vi "_IP Reporter.vi"(4 "ignore Gateway IP?(T)":bool=TRUE, 6 "Load From File(F)":bool, 8 "error in":errorcluster, 9 "notifier":refnum<notifier>, 10 "Init-Information":string, 11 "Setttings":T1={"address"="234.5.6.7", "receiver port"=58432, "Ignore Gateway IP"=TRUE, "HostName"=""}) -> (0 "error out":errorcluster)   [LabVIEW 2017]
doc: "Creates a write-only UDP multicast session and sends data to the specified port."
uses:
  _Typedef/Def-IniSettings -- Cluster.ctl
  _Typedef/Def-Report -- Cluster.ctl
  d1e7c7ed-84d8-4585-9177-9cc17e079b9e.vi
  <vilib>/Utility/error.llb/Clear Errors.vi
  d1e7c7ed-84d8-4585-9177-9cc17e079b9e.vi/c738ad2c-660d-48ef-8aa3-24bba17e300f.vi
  <vilib>/Utility/libraryn.llb/Recursive File List.vi
  <vilib>/Utility/config.llb/Open Config Data.vi
  <userlib>/_OpenG.lib/lvdata/lvdata.llb/Get Data Name__ogtk.vi
  <vilib>/Utility/config.llb/Get Section Names.vi
  <userlib>/_OpenG.lib/variantconfig/variantconfig.llb/Write Section Cluster__ogtk.vi
  <userlib>/_OpenG.lib/variantconfig/variantconfig.llb/Read Section Cluster__ogtk.vi
  <vilib>/Utility/config.llb/Close Config Data.vi
  <vilib>/Utility/tcp.llb/UDP Multicast Write-Only Open.vi
panel:
  out "JSON string":string
  in  "Stop":bool
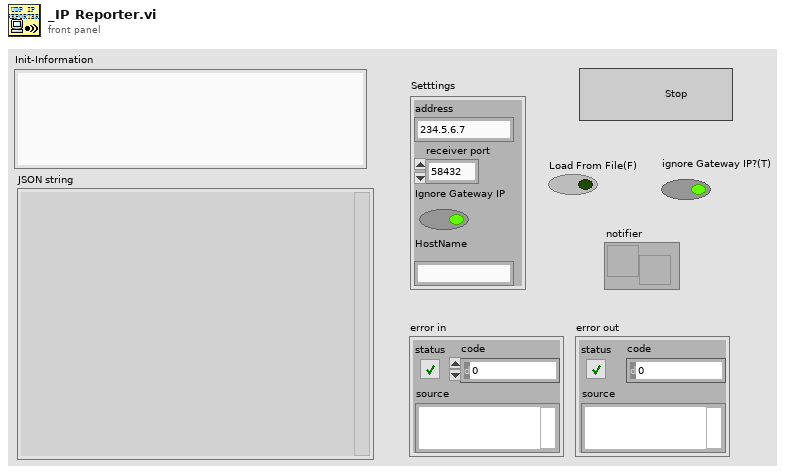
[diagram p1: front panel]
types:
  T1 = typedef "Def-IniSettings -- Cluster.ctl" = cluster{"address":string, "receiver port":u16, "Ignore Gateway IP":bool, "HostName":string}
  T2 = typedef "Def-Report -- Cluster.ctl" = cluster{"Host Name":string, "IPs":string[], "Timestamp":string, "Information":string}
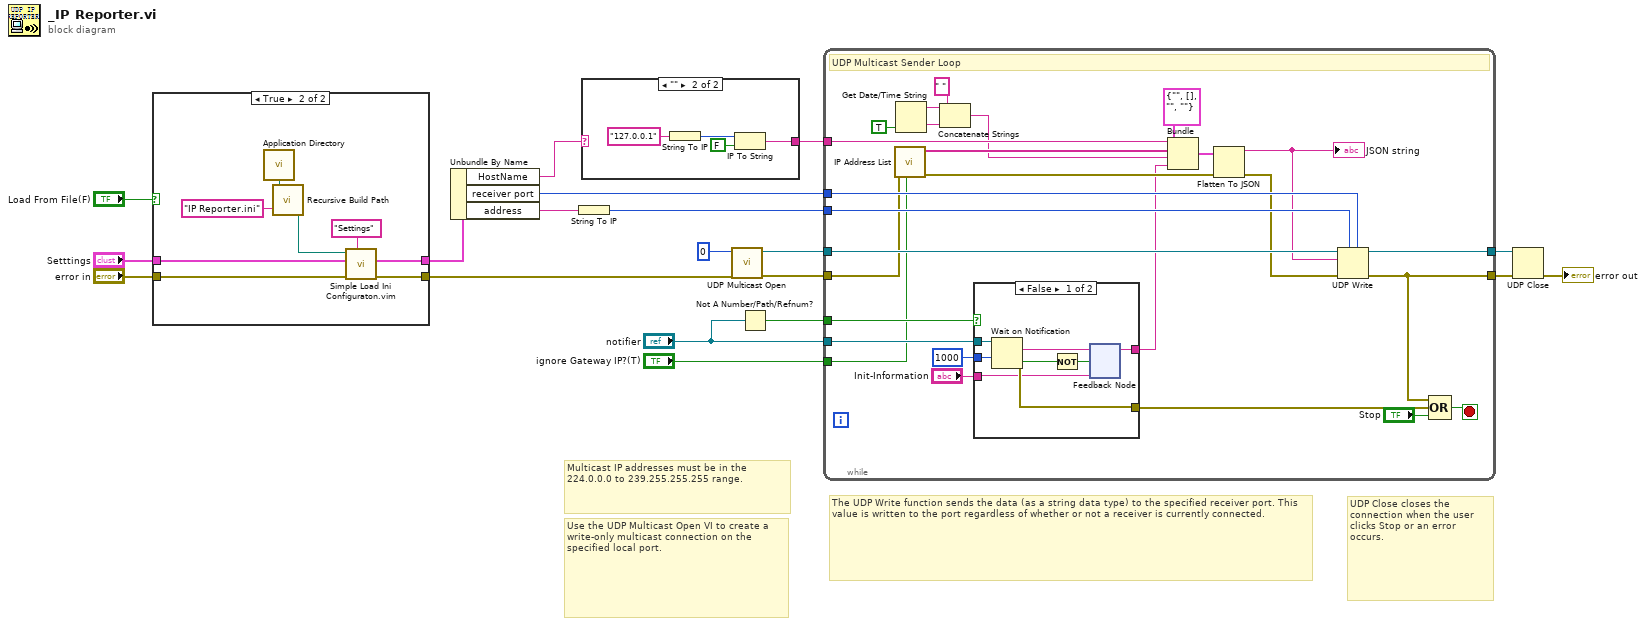
[diagram p0: block diagram]
diagram:
  # "UDP Close closes the connection when the user clicks Stop or an error occurs."
  # "Multicast IP addresses must be in the 224.0.0.0 to 239.255.255.255 range."
  # "The UDP Write function sends the data (as a string data type) to the specified receiver port. This value is written to the port regardless of whether or not a receiver is currently connected."
  # "Use the UDP Multicast Open VI to create a write-only multicast connection on the specified local port."
  n1 = case shown="True" "Load From File(F)" {
    tunnel: [w21 w29] -> w14
    tunnel: [w20 w28] -> w12
    tunnel: "Setttings" -> [w21 w24]
    tunnel: "error in" -> [w20 w23]
    frame False {
    }
    frame True {
      n2 = call <vilib>:"Application Directory.vi"() -> ("Application Directory"=w27:path)
      n3 = call "Recursive Build Path.vi"("file name"="IP Reporter.ini", "Path"=w27) -> ("file path name"=w25:path)  [unwired: 1 in]
      n4 = call "Simple Load Ini Configuraton.vim"("Session"="Settings", "error in (no error)"=w23, "Default Settings"=w24, "file path name"=w25) -> ("error out"=w28:errorcluster, "Settings out"=w29:T1)  [unwired: 6 in]
    }
  }
  n5 = Unbundle By Name(w14) -> ("HostName"=w9:string, "receiver port"=w11:u16, "address"=w13:string)
  n6 = String To IP(1:w13) -> (0:w17:u32)
  n7 = case shown="\"\"" w9 {
    selector: w9 -> [w30 _]
    tunnel: [w30 w34] -> w10
    frame "False", Default {
    }
    frame "" {
      n8 = String To IP(1:"127.0.0.1" ("name")) -> (0:w33:u32)
      n9 = IP To String(1:FALSE ("dot notation? (F)"), 2:w33) -> (0:w34:string)
    }
  }
  n10 = call-poly <vilib>:"UDP Multicast Open.vi"("error in (no error)"=w12, "port"=u16 0) -> ("error out"=w15:errorcluster, "connection ID"=w16:refnum<k16>)  [unwired: 8 in]
  n11 = Not A Number/Path/Refnum?(number/path/refnum="notifier") -> (NaN/Path/Refnum?=w7:bool)
  n12 = while {
    tunnel: [w43] -> w18
    tunnel: w16 -> [w61]
    tunnel: w15 -> [w55]
    tunnel: [w58] -> w19
    tunnel: w17 -> [w57]
    tunnel: w11 -> [w56]
    tunnel: w10 -> [w48]
    tunnel: "notifier" -> [w47]
    tunnel: w7 -> [w44]
    tunnel: "ignore Gateway IP?(T)" -> [w37]
    stop <- w60 stop-if-true
    # "UDP Multicast Sender Loop"
    n13 = call "IP Address List.vi"("ignore Gateway IP?"=w37, "error in (no error)"=w55) -> ("error out"=w54:errorcluster, "Array"=w50:string[])  [unwired: 8 in]
    n14 = Get Date/Time String(want seconds? (F)=TRUE) -> (date string=w42:string, time string=w41:string)  [unwired: 2 in]
    n15 = Concatenate Strings(w42, " " ("string"), w41) -> (w39:string)
    n16 = case shown="False" w44 {
      tunnel: w47 -> [w69 _]
      tunnel: 1000 ("timeout in ms (-1)") -> [w68 _]
      tunnel: [w67 _] -> w45
      tunnel: [w63 w70] -> w36
      tunnel: "Init-Information" -> [w62 w70]
      frame False {
        n17 = Wait on Notification(notifier=w69, timeout in ms (-1)=w68) -> (notification=w65:string, timed out?=w66:bool, error out=w67:errorcluster)  [unwired: 2 in, 1 out]
        n18 = Not(x=w66) -> (.not. x?=w64:bool)
        n19 = feedback-in #1(w65, w64) -> ()
        n20 = feedback #1(w62) -> (w63:string)
      }
      frame True {
      }
    }
    n21 = Bundle(cluster=T2 {"Host Name"="", "IPs"=[], "Timestamp"="", "Information"=""} ("Pack"), "Host Name"=w48, "IPs"=w50, "Timestamp"=w39, "Information"=w36) -> (w49:T2)
    n22 = Flatten To JSON(anything=w49, error in (no error)=w54) -> (JSON string=w52:string, 11:w53:errorcluster)  [unwired: 1 in]
    "JSON string" <- w52
    n23 = UDP Write(address=w57, port or service name=w56, connection ID=w61, data in=w52, 8:w53) -> (error out=w43:errorcluster, 3:w58:refnum<k16>)  [unwired: 1 in]
    n24 = Compound Arithmetic op=OR(w43, w45, "Stop") -> (w60:bool)
  }
  n25 = UDP Close(connection ID=w19, 8:w18) -> (error out=→"error out":errorcluster)  [unwired: 1 out]
